vi "Set Save Settings.vi"(7 "Remove block diagram (true)":bool=TRUE, 8 "error in (no error)":errorcluster, 9 "Remove front panel (true)":bool=TRUE, 10 "ProjectItem Refnum":refnum<vi>, 11 "DLL in":refnum<class "NI_AB_API_DLL.lvclass">) -> (0 "error out":errorcluster, 3 "DLL out":refnum<class "NI_AB_API_DLL.lvclass">)   [LabVIEW 2020, in "NI_AB_API_DLL.lvclass"]
uses:
  <vilib>/AppBuilder/AB_API/DLL/NI_AB_API_DLL.lvclass
  <vilib>/AppBuilder/AB_API/Application/NI_AB_API_Application.lvclass
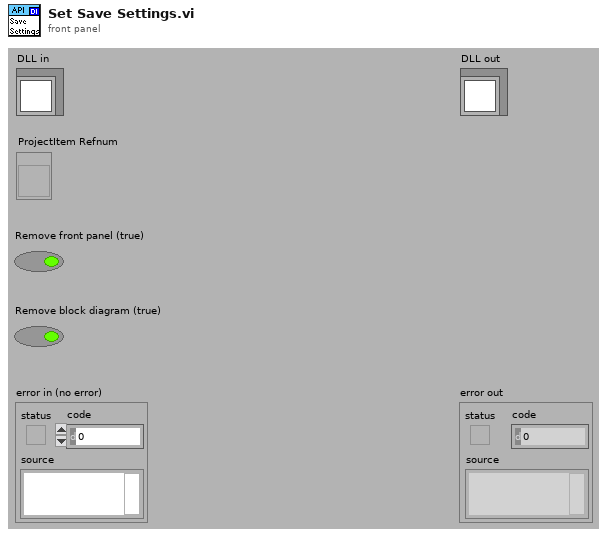
[diagram p1: front panel]
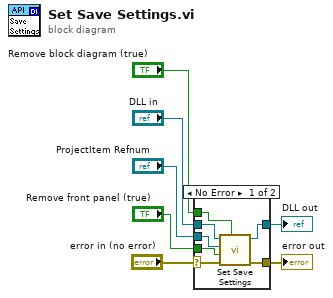
[diagram p0: block diagram]
diagram:
  n1 = case shown="No Error" "error in (no error)" {
    selector: "error in (no error)" -> [w11 w16]
    tunnel: [w12 w16] -> w6
    tunnel: [w13 w15] -> w4
    tunnel: "DLL in" -> [w14 w15]
    tunnel: "ProjectItem Refnum" -> [w8 _]
    tunnel: "Remove block diagram (true)" -> [w10 _]
    tunnel: "Remove front panel (true)" -> [w9 _]
    frame No Error {
      n2 = call-parent "Set Save Settings.vi"("Remove block diagram (true)"=w10, "error in (no error)"=w11, "Remove front panel (true)"=w9, "ProjectItem Refnum"=w8, "NI_AB_API_Build in"=w14) -> ("error out"=w12:errorcluster, "NI_AB_API_Build out"=w13:refnum<class "NI_AB_API_DLL.lvclass">)  [unwired: 5 in]
    }
    frame Error {
    }
  }
  "error out" <- w6
  "DLL out" <- w4
